vi "Alter Value_subVI.vi"(8 "error in (no error)":errorcluster, 9 "String Output":string, 10 "Input":dbl, 11 "VISA Refnum in":refnum<visa-resource-name>) -> (0 "error out":errorcluster, 2 "New Value":dbl, 3 "VISA Refnum out":refnum<visa-resource-name>)   [LabVIEW 2017]
doc: "Returns the current value of a variable over serial, and then alters it and returns the new value."
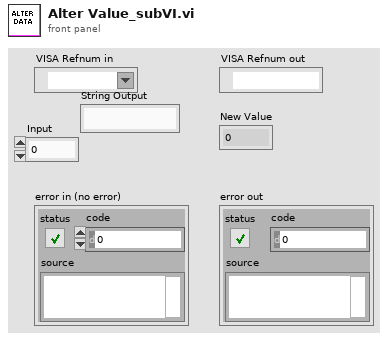
[diagram p1: front panel]
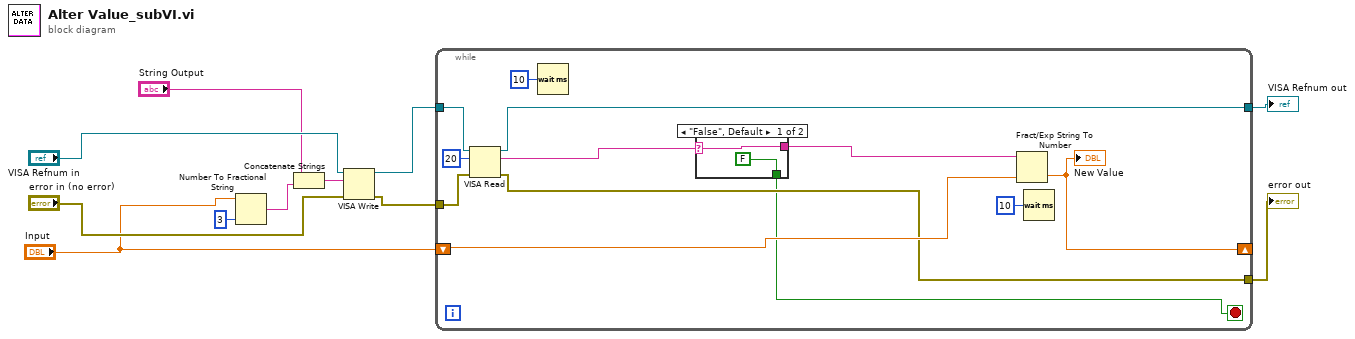
[diagram p0: block diagram]
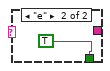
[diagram p2: hidden frame]
diagram:
  n1 = Number To Fractional String(number="Input", precision (6)=i16 3) -> (F-format string=w7:string)  [unwired: 2 in]
  n2 = Concatenate Strings("String Output", w7) -> (w5:string)
  n3 = VISA Write(VISA resource name="VISA Refnum in", write buffer=w5, error in (no error)="error in (no error)") -> (VISA resource name out=w10:refnum<visa-resource-name>, error out=w11:errorcluster)  [unwired: 1 out]
  n4 = while {
    tunnel: w10 -> [w23]
    tunnel: [w21] -> w3
    tunnel: w11 -> [w22]
    tunnel: [w15] -> w4
    shift-right: [w12] -> _
    shift-left: "Input" -> [w16]
    stop <- w14 stop-if-true
    n5 = VISA Read(VISA resource name=w23, byte count=u32 20, error in (no error)=w22) -> (VISA resource name out=w21:refnum<visa-resource-name>, read buffer=w19:string, error out=w15:errorcluster)  [unwired: 1 out]
    n6 = Wait (ms)(milliseconds to wait=u32 10) -> ()  [unwired: 1 out]
    n7 = case shown="\"False\", Default" w19 {
      selector: w19 -> [w25 _]
      tunnel: [FALSE TRUE] -> w14
      tunnel: [w25 _] -> w18
      frame "False", Default {
      }
      frame "e" {
      }
    }
    n8 = Fract/Exp String To Number(string=w18, default (0 dbl)=w16) -> (number=w12:dbl)  [unwired: 2 in, 1 out]
    "New Value" <- w12
    n9 = Wait (ms)(milliseconds to wait=u32 10) -> ()  [unwired: 1 out]
  }
  "error out" <- w4
  "VISA Refnum out" <- w3
